vi "Odometry Loop.vi"(6 "error in (no error)":errorcluster) -> ()   [LabVIEW 2017]
uses:
  <vilib>/Platform/TimedLoop/XDataNode/timing_clust.ctl
  <vilib>/Platform/TimedLoop/XDataNode/nitl_modes.ctl
  <vilib>/Platform/TimedLoop/XDataNode/wakeup.ctl
  Typedef/Odometry.ctl
  Drive/Pure Pursuit/Typedef/Pure Pursuit Telemetry.ctl
  Drive/Pure Pursuit/Typedef/Path Point.ctl
  <vilib>/Analysis/coordinate.llb/2D Cartesian Coordinate Rotation.vi
  <vilib>/Analysis/coordinate.llb/2D Cartesian Coordinate Rotation (Scalar).vi
  <vilib>/Rock Robotics/Network Tables/NT Write Number.vi
  <vilib>/Rock Robotics/Network Tables/NT Write Numeric Array.vi
  Drive/Pure Pursuit/Visualization/Current Path.vi
  <vilib>/Rock Robotics/WPI/ThirdParty/Phoenix-LabVIEW/Motor Controller/Get/CTRE_Phoenix_MotorController_GetVoltage.vi
  <vilib>/Rock Robotics/WPI/ThirdParty/Phoenix-LabVIEW/Motor Controller/Get/CTRE_Phoenix_MotorController_GetSelectedSensorData.vi
  SubVI/OptimizedFPGA_SPI_ReadAuto.vi
  SubVI/WPI_Gyro_ADXRS453_ParseSensorData_Optimized.vi
  <vilib>/platform/TimedLoop/XDataNode/XDataNode.xnode
  <vilib>/Platform/TimedLoop/XDataNode/XDNodeRunTimeDep.lvlib
  Drive/Pure Pursuit/Pure Pursuit.lvlib
panel:
  out "Late Iterations":i16
  out "XY Graph":cluster{dbl[], dbl[]}[](graph)=[{array[1000 elements], array[1000 elements]}, {[-2.247939211922799, 9.450601976465425, 8.114176327244312, -3.5843648611439116, -2.247939211922799], [3.8835413402382706, 1.2106900417960451, -4.638580552398066, -1.9657292539558406, 3.8835413402382706]}, {[0.0, 40.0, 60.0, 100.0], [0.0, 20.0, 80.0, 40.0]}, {array[304 elements], array[304 elements]}, {[7.524752475247524, 1.9801980198019802], [-4.118238955689372, -1.1545613507952672]}, {[-5.727080057823512, -5.705598316147173, -5.641285533198998, -5.534538218672029, -5.386014505257412, -5.196630091037495, -4.967552593902651, -4.700194352798713, -4.396203720187724, -4.057454899406876, -3.686036389581695, -3.28423810933444, -2.8545372786743237, -2.3995831461123918, -1.922180655163488, -1.4252731509367513, -0.9119242334342519, -0.38529886943823066, 0.15135612056157366, 0.6947320800959187, 1.241478915683433, 1.7882257512709472, 2.331601710805292, 2.8682567008050963, 3.3948820648011178, 3.9082309823036177, 4.405138486530354, 4.882540977479257, 5.337495110041189, 5.767195940701306, 6.16899422094856, 6.540412730773742, 6.87916155155459, 7.1831521841655785, 7.450510425269517, 7.679587922404362, 7.86897233662428, 8.017496050038897, 8.124243364565864, 8.18855614751404, 8.210037889190378, 8.18855614751404, 8.124243364565865, 8.017496050038897, 7.86897233662428, 7.679587922404362, 7.450510425269517, 7.18315218416558, 6.879161551554592, 6.540412730773744, 6.168994220948562, 5.76719594070131, 5.337495110041191, 4.882540977479256, 4.405138486530356, 3.9082309823036216, 3.3948820648011195, 2.868256700805095, 2.3316017108052938, 1.788225751270952, 1.2414789156834347, 0.6947320800959172, 0.15135612056157544, -0.3852988694382258, -0.9119242334342501, -1.4252731509367527, -1.9221806551634866, -2.3995831461123878, -2.854537278674323, -3.2842381093344417, -3.686036389581693, -4.057454899406872, -4.396203720187724, -4.700194352798713, -4.967552593902649, -5.196630091037493, -5.386014505257412, -5.534538218672031, -5.641285533198998, -5.705598316147173, -5.727080057823512], [-7.13175642584397, -7.6785032614314845, -8.22187922096583, -8.758534210965633, -9.285159574961655, -9.798508492464155, -10.295415996690892, -10.772818487639794, -11.227772620201726, -11.657473450861843, -12.059271731109098, -12.430690240934279, -12.769439061715127, -13.073429694326116, -13.340787935430054, -13.5698654325649, -13.759249846784815, -13.907773560199434, -14.0145208747264, -14.078833657674576, -14.100315399350915, -14.078833657674576, -14.0145208747264, -13.907773560199434, -13.759249846784817, -13.5698654325649, -13.340787935430054, -13.073429694326116, -12.769439061715127, -12.430690240934279, -12.0592717311091, -11.657473450861843, -11.227772620201728, -10.772818487639796, -10.295415996690892, -9.798508492464155, -9.285159574961655, -8.758534210965635, -8.22187922096583, -7.678503261431485, -7.131756425843971, -6.5850095902564565, -6.041633630722112, -5.504978640722308, -4.978353276726287, -4.465004359223786, -3.9680968549970497, -3.4906943640481467, -3.035740231486214, -2.6060394008260976, -2.2042411205788426, -1.8328226107536638, -1.4940737899728127, -1.1900831573618227, -0.922724916257887, -0.6936474191230433, -0.504263004903124, -0.355739291488506, -0.2489919769615394, -0.18467919401336363, -0.16319745233702498, -0.18467919401336363, -0.24899197696153852, -0.355739291488506, -0.5042630049031231, -0.6936474191230424, -0.9227249162578861, -1.1900831573618218, -1.4940737899728118, -1.832822610753662, -2.2042411205788417, -2.6060394008260923, -3.035740231486211, -3.4906943640481467, -3.9680968549970475, -4.465004359223782, -4.978353276726283, -5.5049786407223085, -6.041633630722109, -6.585009590256451, -7.131756425843968]}]
  out "Drivetrain Chart":T1(graph)
  out "Gyro":dbl(graph)
  out "Encoders":T2(graph)
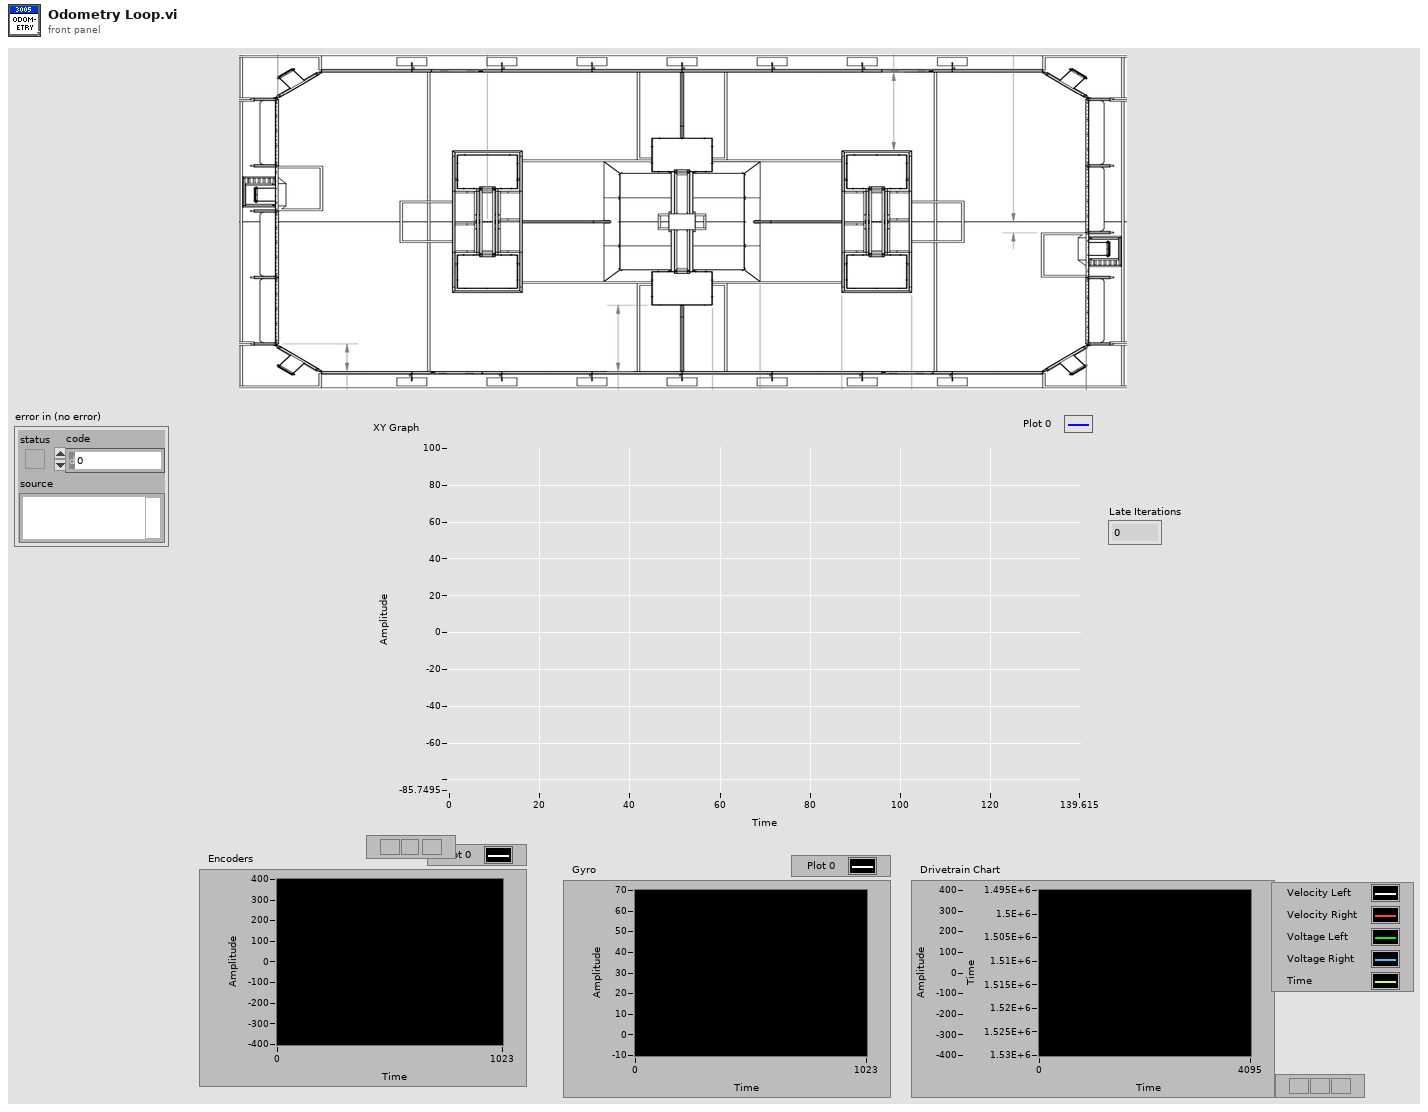
[diagram p1: front panel]
types:
  T1 = cluster{"Left Velocity Raw":i32, "Right Velocity Raw":i32, "Output Voltage":dbl, "Output Voltage":dbl, "Tick Count(mSec)":u32}
  T2 = cluster{"Left Velocity Raw":i32, "Right Velocity Raw":i32}
  T3 = typedef "TalonSRX6Motor.ctl" = cluster{"FrontLeftMaster":T4, "FrontLeftSlave1":T4, "FrontLeftSlave2":T4, "FrontRightMaster":T4, "FrontRightSlave1":T4, "FrontRightSlave2":T4}
  T4 = typedef "WPI_MotorControlDeviceRef.ctl" = cluster{"DeviceStatus":errorcluster, "Type":T5, "PWM":cluster{"PWM Channel":T6, "DeadBand":T7}, "CAN":cluster{"Device Number":u8, "SetOutput VI Ref":variant, "GetOutput VI Ref":variant, "Enable VI Ref":variant, "Disable VI Ref":variant, "Data":variant}, "Invert":bool, "DIO PWM":cluster{"PWM \"Enable\" Channel":T6, "DIOChannel":T8, "PWM Rate":dbl}}
  T5 = typedef "WPI_MotorControlType.ctl" = enum16{"PWM", "CAN", "DIO PWM"}
  T6 = typedef "FPGA_DIOPWMChannel.ctl" = enum8{"PWM 0", "PWM 1", "PWM 2", "PWM 3", "PWM 4", "PWM 5", "PWM 6", "PWM 7", "PWM 8", "PWM 9", "PWM MXP 0", "PWM MXP 1", "PWM MXP 2", "PWM MXP 3", "PWM MXP 4", "PWM MXP 5", "PWM MXP 6", "PWM MXP 7", "PWM MXP 8", "PWM MXP 9", "Invalid"}
  T7 = typedef "WPI_PWMDeadband.ctl" = cluster{"Name":string, "maxPositivePwm":i32, "minPositivePwm":i32, "centerPwm":i32, "maxNegativePwm":i32, "minNegativePwm":i32, "angularRange":u16}
  T8 = typedef "FPGA_DIOChannel.ctl" = enum8{"DIO 0", "DIO 1", "DIO 2", "DIO 3", "DIO 4", "DIO 5", "DIO 6", "DIO 7", "DIO 8", "DIO 9", "DIO MXP 0", "DIO MXP 1", "DIO MXP 2", "DIO MXP 3", "DIO MXP 4", "DIO MXP 5", "DIO MXP 6", "DIO MXP 7", "DIO MXP 8", "DIO MXP 9", "DIO MXP 10", "DIO MXP 11", "DIO MXP 12", "DIO MXP 13", "DIO MXP 14", "DIO MXP 15", "SPI Port CS1", "SPI Port CS2", "SPI Port CS3", "SPI Port MISO", "SPI Port MOSI", "Invalid"}
  T9 = typedef "XDNodeRunTimeDep.lvlib/timing_clust.ctl" = cluster{"Expected End [f-1]":u64, "Actual End [f-1]":u64, "Finished Late? [f-1]":bool, "Expected End [i-1]":u64, "Actual End [i-1]":u64, "Finished Late? [i-1]":bool, "Expected Start [i]":u64, "Actual Start [i]":u64, "Expected Start [f]":u64, "Actual Start [f]":u64, "Source Name":string, "Structure Name":string, "Period":i64, "Deadline":i64, "Offset":i64, "Start":i64, "Priority":i32, "Timeout":i32, "Mode":T10, "Wakeup Reason":T11, "Error":errorcluster, "Source Type":string, "Secondary Source Type":string, "Global End Time":u64, "Global Start Time":u64, "Frame Duration":u64, "Iteration Duration":u64, "Assigned CPU":i32, "I/O Scan Engine Mode":u32}
  T10 = typedef "XDNodeRunTimeDep.lvlib/nitl_modes.ctl" = enum32{"No Change", "Process missed periods, maintain original phase", "Discard missed periods, maintain original phase", "Process missed periods, ignore original phase", "Discard missed periods, ignore original phase"}
  T11 = typedef "XDNodeRunTimeDep.lvlib/wakeup.ctl" = enum32{"Normal", "Aborted", "Asynchronous wakeup", "Timing source error", "Timed loop error", "Timeout"}
  T12 = typedef "WPI_GyroDevRef.ctl" = cluster{"DevStatus":errorcluster, "Analog Channel":T13, "Gain (VoltsPerDegree/Second)":dbl, "Gyro Type":enum16{"Analog", "XRS450"}, "Handle":i32, "SPI Bus":T14, "Device Found":bool, "Sample Rate":dbl, "Calibrate On Open":bool, "Offset":dbl}
  T13 = typedef "FPGA_AIChannel.ctl" = enum8{"AI 0", "AI 1", "AI 2", "AI 3", "AI MXP 0", "AI MXP 1", "AI MXP 2", "AI MXP 3", "Invalid"}
  T14 = typedef "spi_bus.ctl" = enum16{"SPI On-Board, CS0", "SPI On-Board, CS1", "SPI On-Board, CS2", "SPI On-Board, CS3", "SPI MXP", "Invalid"}
  T15 = typedef "Odometry.ctl" = cluster{"x":dbl, "y":dbl, "theta":dbl, "Left Encoder Raw":i32, "Right Encoder Raw":i32, "Left Velocity Raw":i32, "Right Velocity Raw":i32, "Left Encoder":dbl, "Right Encoder":dbl, "Late Iterations":i16}
  T16 = typedef "Pure Pursuit.lvlib/Pure Pursuit Telemetry.ctl" = cluster{"Target Point":T17, "Close Point":T17, "Curvature":dbl, "index out":i32}
  T17 = typedef "Pure Pursuit.lvlib/Path Point.ctl" = cluster{"x":dbl, "y":dbl, "heading":dbl, "curvature":dbl, "total distance":dbl, "velocity expected":dbl}
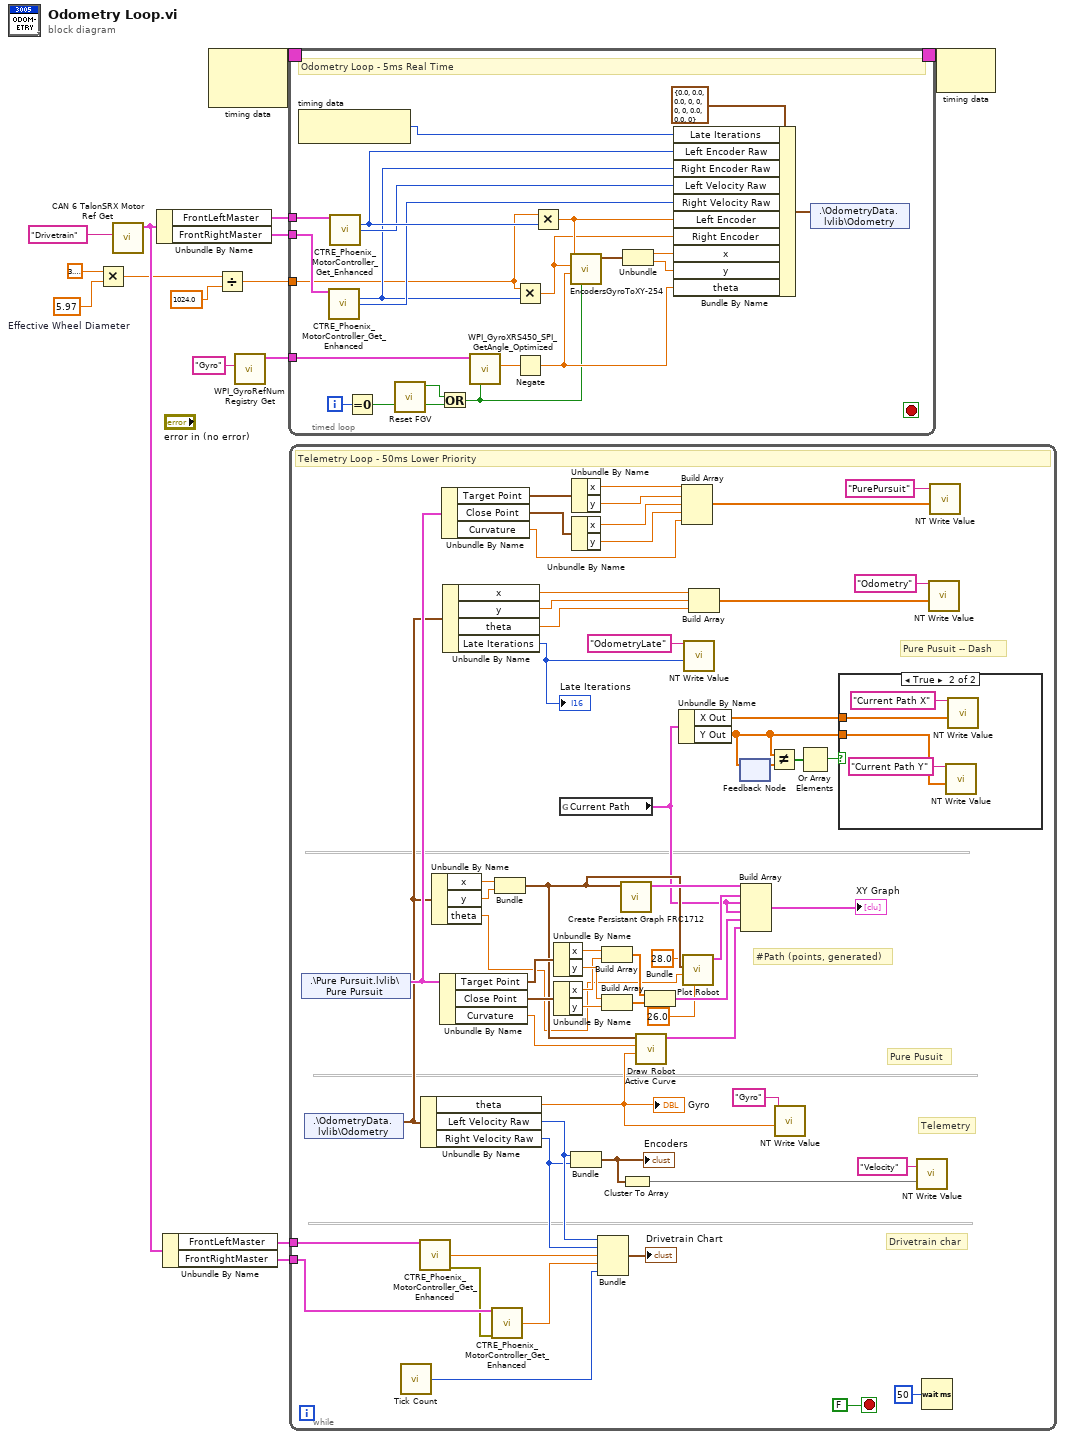
[diagram p0: block diagram]
diagram:
  w5 = 5.97  # Effective Wheel Diameter
  n1 = Multiply(x=3.141592653589793, y=w5) -> (x*y=w3:dbl)
  n2 = call "CAN 6 TalonSRX Motor Ref Get.vi"("refnum name"="Drivetrain") -> ("TalonSRX6MotorRef out"=w8:T3)  [unwired: 9 in, 1 out]
  n3 = Unbundle By Name(w8) -> ("FrontLeftMaster"=w12:T4, "FrontRightMaster"=w13:T4)
  n4 = Unbundle By Name(w8) -> ("FrontLeftMaster"=w7:T4, "FrontRightMaster"=w6:T4)
  n5 = node-c288() -> (w15:T9)  [unwired: 2 in]
  n6 = Divide(x=w3, y=1024.0) -> (x/y=w1:dbl)
  n7 = call <vilib>:"WPI_GyroRefNum Registry Get.vi"("refnum name"="Gyro") -> ("GyroDevRef"=w10:T12)  [unwired: 9 in, 1 out]
  n8 = timed-loop {
    timing: w15 -> [_]
    timing-out: [_] -> w14
    tunnel: w10 -> [w23]
    tunnel: w12 -> [w37]
    tunnel: w13 -> [w36]
    tunnel: w1 -> [w20]
    i -> [w35]
    stop <- _ stop-if-true
    # "Odometry Loop - 5ms Real Time"
    n9 = node-c288() -> (w16:i64)  [unwired: 1 in]
    n10 = call-poly <vilib>:"CTRE_Phoenix_MotorController_Get_Enhanced.vi"("PhoenixMotorControlDevRef"=w36) -> ("Position (Raw Sensor Units)"=w21:i32, "Velocity (Raw Sensor Units per 100 ms)"=w24:i32)  [unwired: 11 in, 2 out]
    n11 = call-poly <vilib>:"CTRE_Phoenix_MotorController_Get_Enhanced.vi"("PhoenixMotorControlDevRef"=w37) -> ("Position (Raw Sensor Units)"=w26:i32, "Velocity (Raw Sensor Units per 100 ms)"=w25:i32)  [unwired: 11 in, 2 out]
    n12 = Equal To 0?(x=w35) -> (x = 0?=w18:bool)
    n13 = call "Reset FGV.vi"() -> ("Reset?"=w19:bool)  [unwired: 11 in]
    n14 = Or(x=w19, y=w18) -> (x .or. y?=w17:bool)
    n15 = call "WPI_GyroXRS450_SPI_GetAngle_Optimized.vi"("Reset?"=w17, "GyroDevRef"=w23) -> ("Angle"=w22:dbl)  [unwired: 6 in, 3 out]
    n16 = Multiply(x=w20, y=w21) -> (x*y=w27:dbl)
    n17 = Negate(x=w22) -> (-x=w30:dbl)
    n18 = Multiply(x=w20, y=w26) -> (x*y=w28:dbl)
    n19 = call "EncodersGyroToXY-254.vi"("Reset"=w17, "Angle (degrees)"=w30, "Right Distance"=w27, "Left Distance"=w28) -> ("Location"=w33:cluster{"X":dbl, "Y":dbl})  [unwired: 7 in]
    n20 = Unbundle(w33) -> ("X"=w32:dbl, "Y"=w31:dbl)
    n21 = Bundle By Name(cluster=T15 {"x"=0.0, "y"=0.0, "theta"=0.0, "Left Encoder Raw"=0, "Right Encoder Raw"=0, "Left Velocity Raw"=0, "Right Velocity Raw"=0, "Left Encoder"=0.0, "Right Encoder"=0.0, "Late Iterations"=0} ("Odometry"), "Late Iterations"=w16, "Left Encoder Raw"=w26, "Right Encoder Raw"=w21, "Left Velocity Raw"=w25, "Right Velocity Raw"=w24, "Left Encoder"=w28, "Right Encoder"=w27, "x"=w32, "y"=w31, "theta"=w30) -> (w29:T15)
    n22 = shared-variable ".\\OdometryData.lvlib\\Odometry"(w29) -> ()  [unwired: 1 in, 1 out]
  }
  n23 = while {
    tunnel: w7 -> [w96]
    tunnel: w6 -> [w95]
    stop <- FALSE stop-if-true
    # "Pure Pusuit -- Dash"
    # "Telemetry"
    # "Drivetrain char"
    # "Pure Pusuit"
    # "#Path (points, generated)"
    # "Telemetry Loop - 50ms Lower Priority"
    n24 = shared-variable ".\\Pure Pursuit.lvlib\\Pure Pursuit"() -> (w62:T16)  [unwired: 1 in, 1 out]
    n25 = shared-variable ".\\OdometryData.lvlib\\Odometry"() -> (w53:T15)  [unwired: 1 in, 1 out]
    n26 = call "Tick Count"() -> ("Tick Count(mSec)"=w69:u32)
    n27 = call-poly <vilib>:"CTRE_Phoenix_MotorController_Get_Enhanced.vi"("PhoenixMotorControlDevRef"=w96) -> ("Output Voltage"=w92:dbl, "error out"=w63:errorcluster)  [unwired: 10 in, 3 out]
    n28 = Unbundle By Name(w53) -> ("theta"=w74:dbl, "Left Velocity Raw"=w94:i32, "Right Velocity Raw"=w93:i32)
    "Gyro" <- w74
    n29 = Unbundle By Name(w53) -> ("x"=w89:dbl, "y"=w88:dbl, "theta"=w71:dbl)
    n30 = Unbundle By Name(w62) -> ("Target Point"=w78:T17, "Close Point"=w77:T17, "Curvature"=w76:dbl)
    n31 = Unbundle By Name(w62) -> ("Target Point"=w61:T17, "Close Point"=w60:T17, "Curvature"=w55:dbl)
    n32 = Unbundle By Name(w53) -> ("x"=w52:dbl, "y"=w51:dbl, "theta"=w50:dbl, "Late Iterations"=w41:i16)
    "Late Iterations" <- w41
    n33 = call-poly <vilib>:"CTRE_Phoenix_MotorController_Get_Enhanced.vi"("PhoenixMotorControlDevRef"=w95, "error in"=w63) -> ("Output Voltage"=w91:dbl)  [unwired: 9 in, 4 out]
    n34 = Bundle("x"=w89, "y"=w88) -> (w73:cluster{"x":dbl, "y":dbl})  [unwired: 1 in]
    n35 = Unbundle By Name(w78) -> ("x"=w85:dbl, "y"=w84:dbl)
    n36 = Unbundle By Name(w77) -> ("x"=w81:dbl, "y"=w80:dbl)
    n37 = global read "Current Path.vi" "Current Path"() -> (w48:cluster{"X Out":dbl[], "Y Out":dbl[]})
    n38 = Bundle("Left Velocity Raw"=w94, "Right Velocity Raw"=w93) -> (w67:T2)  [unwired: 1 in]
    "Encoders" <- w67
    n39 = Unbundle By Name(w61) -> ("x"=w59:dbl, "y"=w58:dbl)
    n40 = Unbundle By Name(w60) -> ("x"=w57:dbl, "y"=w56:dbl)
    n41 = Bundle("Left Velocity Raw"=w94, "Right Velocity Raw"=w93, "Output Voltage"=w92, "Output Voltage"=w91, "Tick Count(mSec)"=w69) -> (→"Drivetrain Chart":T1)  [unwired: 1 in]
    n42 = Build Array(w85, w81) -> (w82:dbl[])
    n43 = Build Array(w84, w80) -> (w83:dbl[])
    n44 = call "Create Persistant Graph FRC1712.vi"("XY"=w73) -> ("Graph Plot"=w98:cluster{dbl[], dbl[]})  [unwired: 10 in]
    n45 = Cluster To Array(cluster=w67) -> (array=w66:i32[])
    n46 = call "Draw Robot Active Curve.vi"("theta"=w74, "Curvature"=w76, "Cluster"=w73) -> ("circle"=w75:cluster{dbl[], dbl[]})  [unwired: 8 in]
    n47 = Bundle(w82, w83) -> (w79:cluster{dbl[], dbl[]})  [unwired: 1 in]
    n48 = Unbundle By Name(w48) -> ("X Out"=w47:dbl[], "Y Out"=w45:dbl[])
    n49 = Build Array(w59, w58, w57, w56, w55) -> (w54:dbl[])
    n50 = call "Plot Robot.vi"("Length"=26.0, "Angle"=w71, "Location"=w73, "Width"=28.0) -> ("Cluster"=w86:cluster{"X Out":dbl[], "Y Out":dbl[]})  [unwired: 7 in]
    n51 = call-poly <vilib>:"NT Write Value.vi"("Numeric"=w41, "Name"="OdometryLate") -> ()  [unwired: 9 in, 1 out]
    n52 = Build Array(w52, w51, w50) -> (w49:dbl[])
    n53 = feedback-in #1(w45) -> ()
    n54 = feedback #1() -> (w46:dbl[])  [unwired: 1 in]
    n55 = Build Array(w98, w86, w48, w48, w79, w75) -> (→"XY Graph":cluster{"X Out":dbl[], "Y Out":dbl[]}[])
    n56 = Not Equal?(x=w45, y=w46) -> (x != y?=w44:bool[])
    n57 = call-poly <vilib>:"NT Write Value.vi"("Numeric"=w74, "Name"="Gyro") -> ()  [unwired: 9 in, 1 out]
    n58 = Or Array Elements(Boolean array=w44) -> (logical OR=w43:bool)
    n59 = case shown="True" w43 {
      tunnel: w45 -> [_ w102]
      tunnel: w47 -> [_ w101]
      frame False {
      }
      frame True {
        n60 = call-poly <vilib>:"NT Write Value.vi"("Numeric Array"=w102, "Name"="Current Path Y") -> ()  [unwired: 9 in, 1 out]
        n61 = call-poly <vilib>:"NT Write Value.vi"("Numeric Array"=w101, "Name"="Current Path X") -> ()  [unwired: 9 in, 1 out]
      }
    }
    n62 = call-poly <vilib>:"NT Write Value.vi"("Numeric Array"=w66, "Name"="Velocity") -> ()  [unwired: 9 in, 1 out]
    n63 = Wait (ms)(milliseconds to wait=u32 50) -> ()  [unwired: 1 out]
    n64 = call-poly <vilib>:"NT Write Value.vi"("Numeric Array"=w49, "Name"="Odometry") -> ()  [unwired: 9 in, 1 out]
    n65 = call-poly <vilib>:"NT Write Value.vi"("Numeric Array"=w54, "Name"="PurePursuit") -> ()  [unwired: 9 in, 1 out]
  }
  n66 = node-c288(w14) -> ()  [unwired: 1 out]
